vi "SeCrTs-NS Main.vi"(8 "error in (no error)":errorcluster, 9 "Selct type":enum16{"Both", "Pump", "Storage"}(ring)=enum."Pump", 10 "Pumb Ip Address":string, 11 "Storage Ip Address":string) -> (0 "error out":errorcluster, 2 "Pumb Connected  ?":bool, 3 "Storage Connected  ?":bool)   [LabVIEW 2022 SP3]
uses:
  Controls/SeCrTs-NS Data type.ctl
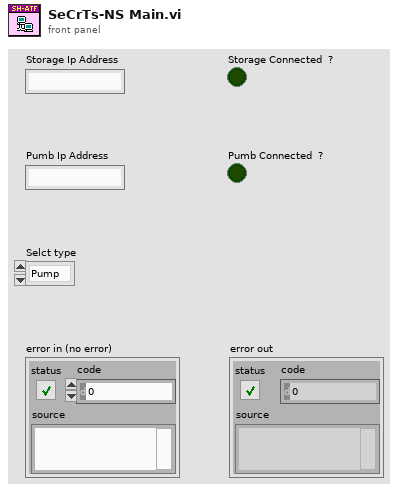
[diagram p1: front panel]
types:
  T1 = typedef "SeCrTs-NS Data type.ctl" = cluster{"DI_Data":digitalwaveform[], "Drive_A_C":waveform(dbl)[], "Drive_A_D":waveform(dbl)[], "Drive_L_C":waveform(dbl)[], "Drive_L_D":waveform(dbl)[], "Loop Status":bool[], "CDT":dbl, "RT Error":cluster{"Error Code":string, "Error Source":string}, "DO":waveform(dbl)[], "SEQ Monitor":string[], "Device List":string}
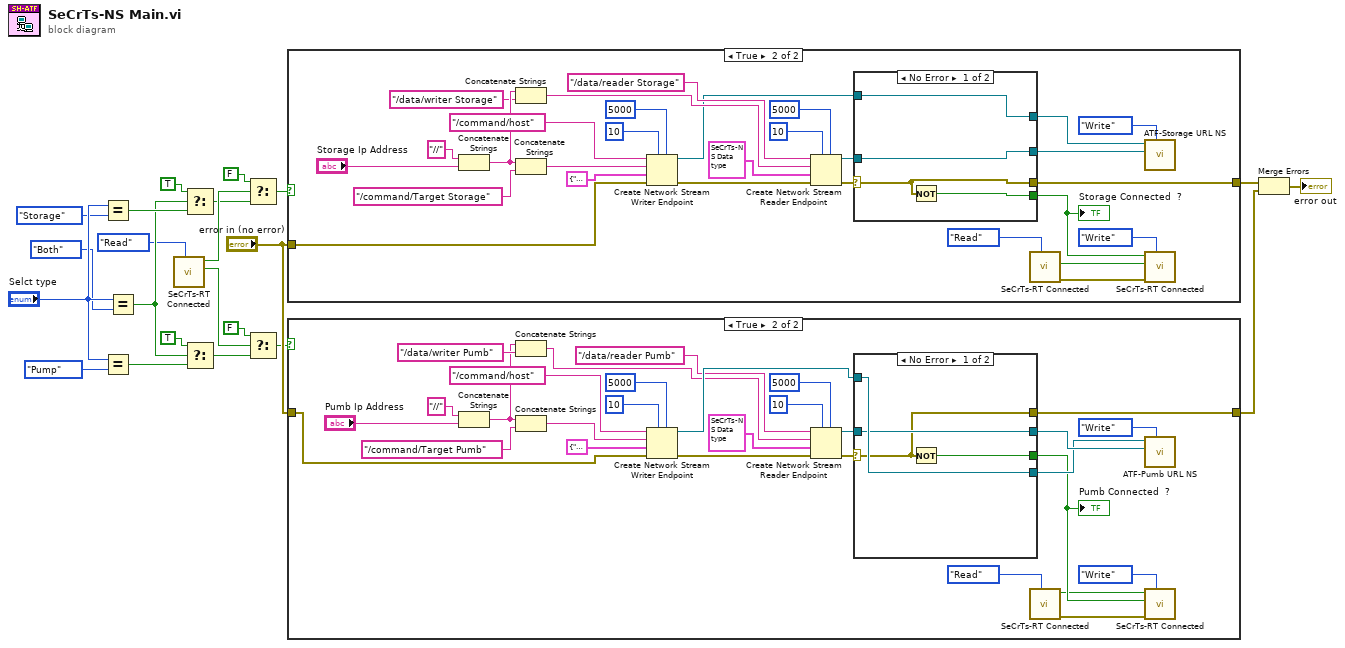
[diagram p0: block diagram]
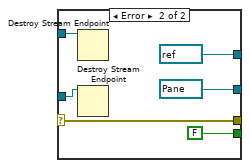
[diagram p3: hidden frame]
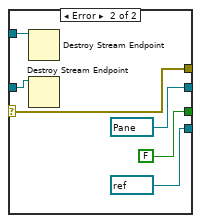
[diagram p5: hidden frame]
diagram:
  n1 = Equal?(x="Selct type", y=enum16{"Both", "Pump", "Storage"}."Storage" ("Selct type 2")) -> (x = y?=w16:bool)
  n2 = Equal?(x="Selct type", y=enum16{"Both", "Pump", "Storage"}."Pump" ("Selct type 2")) -> (x = y?=w13:bool)
  n3 = Equal?(x="Selct type", y=enum16{"Both", "Pump", "Storage"}."Both" ("Selct type 2")) -> (x = y?=w14:bool)
  n4 = call "SeCrTs-RT Connected .vi"("Enum"=enum16{"Read", "Write"}."Read") -> ("Pumb rt con R"=w6:bool, "Stoarge rt con R"=w11:bool)  [unwired: 8 in, 1 out]
  n5 = Select(t=TRUE, s=w14, f=w16) -> (s? t:f=w9:bool)
  n6 = Select(t=TRUE, s=w14, f=w13) -> (s? t:f=w5:bool)
  n7 = Select(t=FALSE, s=w11, f=w9) -> (s? t:f=w8:bool)
  n8 = Select(t=FALSE, s=w6, f=w5) -> (s? t:f=w4:bool)
  n9 = case shown="True" w8 {
    tunnel: [w23 w36] -> w20
    tunnel: "error in (no error)" -> [w23 w32]
    frame False {
    }
    frame True {
      n10 = Concatenate Strings("//" ("reader url"), "Storage Ip Address") -> (w50:string)
      n11 = Concatenate Strings(w50, "/data/writer Storage" ("reader url")) -> (w45:string)
      n12 = Concatenate Strings(w50, "/command/Target Storage" ("reader url")) -> (w46:string)
      n13 = Create Network Stream Writer Endpoint(5:5000 ("timeout in ms (-1)"), 7:10 ("timeout in ms (-1)"), 8:w32, 9:cluster{"Message":string, "Data":variant} {"Message"="", "Data"=variant}, 10:w46, 11:"/command/host" ("writer name")) -> (0:w43:errorcluster, 3:w38:refnum<k21>)  [unwired: 1 in]
      n14 = Create Network Stream Reader Endpoint(5:5000 ("timeout in ms (-1)"), 7:10 ("reader buffer size"), 8:w43, 9:T1 {"DI_Data"=[], "Drive_A_C"=[], "Drive_A_D"=[], "Drive_L_C"=[], "Drive_L_D"=[], "Loop Status"=[], "CDT"=0.0, "RT Error"={"Error Code"="", "Error Source"=""}, "DO"=[], "SEQ Monitor"=[], "Device List"=""}, 10:w45, 11:"/data/reader Storage" ("writer name")) -> (0:w39:errorcluster, 3:w37:refnum<k21>)  [unwired: 1 in]
      n15 = case shown="No Error" w39 {
        selector: w39 -> [w54 w59]
        tunnel: [w56 refnum<k21> refnum ("writer name")] -> w30
        tunnel: w38 -> [w56 w62]
        tunnel: [w55 refnum<k21> refnum ("writer name")] -> w31
        tunnel: w37 -> [w55 w61]
        tunnel: [w54 w59] -> w36
        tunnel: [w53 FALSE] -> w25
        frame No Error {
          n16 = Not(x=w54) -> (.not. x?=w53:bool)
        }
        frame Error {
          n17 = Destroy Stream Endpoint(11:w62) -> ()  [unwired: 1 in, 1 out]
          n18 = Destroy Stream Endpoint(11:w61) -> ()  [unwired: 1 in, 1 out]
        }
      }
      "Storage Connected  ?" <- w25
      n19 = call "SeCrTs-RT Connected .vi"("Enum"=enum16{"Read", "Write"}."Read") -> ("error out"=w26:errorcluster, "Pumb rt con R"=w24:bool)  [unwired: 8 in, 1 out]
      n20 = call "ATF-Storage URL NS.vi"("Enum"=enum16{"Init", "Read", "Write"}."Write", "Storage Reader"=w31, "Storage writer url"=w30) -> ()  [unwired: 7 in, 2 out]
      n21 = call "SeCrTs-RT Connected .vi"("Enum"=enum16{"Read", "Write"}."Write", "error in"=w26, "Pumb rt con"=w24, "Storage rt con"=w25) -> ()  [unwired: 5 in, 3 out]
    }
  }
  n22 = case shown="True" w4 {
    tunnel: "error in (no error)" -> [w63 w73]
    tunnel: [w63 w72] -> w19
    frame False {
    }
    frame True {
      n23 = Concatenate Strings("//" ("reader url"), "Pumb Ip Address") -> (w76:string)
      n24 = Concatenate Strings(w76, "/data/writer Pumb" ("reader url")) -> (w81:string)
      n25 = Concatenate Strings(w76, "/command/Target Pumb" ("reader url")) -> (w80:string)
      n26 = Create Network Stream Writer Endpoint(5:5000 ("timeout in ms (-1)"), 7:10 ("timeout in ms (-1)"), 8:w73, 9:cluster{"Message":string, "Data":variant} {"Message"="", "Data"=variant}, 10:w80, 11:"/command/host" ("writer name")) -> (0:w83:errorcluster, 3:w88:refnum<k21>)  [unwired: 1 in]
      n27 = Create Network Stream Reader Endpoint(5:5000 ("timeout in ms (-1)"), 7:10 ("reader buffer size"), 8:w83, 9:T1 {"DI_Data"=[], "Drive_A_C"=[], "Drive_A_D"=[], "Drive_L_C"=[], "Drive_L_D"=[], "Loop Status"=[], "CDT"=0.0, "RT Error"={"Error Code"="", "Error Source"=""}, "DO"=[], "SEQ Monitor"=[], "Device List"=""}, 10:w81, 11:"/data/reader Pumb" ("writer name")) -> (0:w87:errorcluster, 3:w89:refnum<k21>)  [unwired: 1 in]
      n28 = case shown="No Error" w87 {
        selector: w87 -> [w94 w99]
        tunnel: [w96 refnum<k21> refnum ("writer name")] -> w69
        tunnel: w88 -> [w96 w102]
        tunnel: [w95 refnum<k21> refnum ("writer name")] -> w70
        tunnel: w89 -> [w95 w101]
        tunnel: [w94 w99] -> w72
        tunnel: [w93 FALSE] -> w66
        frame No Error {
          n29 = Not(x=w94) -> (.not. x?=w93:bool)
        }
        frame Error {
          n30 = Destroy Stream Endpoint(11:w102) -> ()  [unwired: 1 in, 1 out]
          n31 = Destroy Stream Endpoint(11:w101) -> ()  [unwired: 1 in, 1 out]
        }
      }
      "Pumb Connected  ?" <- w66
      n32 = call "SeCrTs-RT Connected .vi"("Enum"=enum16{"Read", "Write"}."Read") -> ("error out"=w64:errorcluster, "Stoarge rt con R"=w65:bool)  [unwired: 8 in, 1 out]
      n33 = call "ATF-Pumb URL NS.vi"("Enum"=enum16{"Init", "Read", "Write"}."Write", "Pumb Reader url"=w70, "Pumb writer"=w69) -> ()  [unwired: 7 in, 2 out]
      n34 = call "SeCrTs-RT Connected .vi"("Enum"=enum16{"Read", "Write"}."Write", "error in"=w64, "Pumb rt con"=w66, "Storage rt con"=w65) -> ()  [unwired: 5 in, 3 out]
    }
  }
  n35 = Merge Errors(w20, w19) -> (→"error out":errorcluster)
